vi "AM Init PS Scan.vi"(8 "error in (no error)":errorcluster, 10 "Message Data":variant, 11 "Hardware Resources in":T1 {"PS Measure Plan" items=["Pretreatment settings (PS)", "Linear Sweep Voltammetry (LSV)", "Differential Pulse Voltammetry (DPV)", "Cyclic Voltammetry (CV)", "Chronoamperometry (CA)", "Chronopotentiometry (CP)", "El Imp Spectroscopy (EIS)"]; "System Preset"."Test Configuration"."SP List" format="%#.1g"}) -> (0 "error out":errorcluster, 3 "Hardware Resources out":T1 {"PS Measure Plan" items=["Pretreatment settings (PS)", "Linear Sweep Voltammetry (LSV)", "Differential Pulse Voltammetry (DPV)", "Cyclic Voltammetry (CV)", "Chronoamperometry (CA)", "Chronopotentiometry (CP)", "El Imp Spectroscopy (EIS)"]; "System Preset"."Test Configuration"."SP List" format="%#.1g"})   [LabVIEW 2020, in "Test Driver.lvlib"]
doc: "Initialize the hardware references."
uses:
  Test Driver.lvlib
  Test Driver Configuration.ctl
  support/Message Queue/Message Cluster.ctl
  System Preset.ctl
  Test Type.ctl
  support/Message Queue/Message Queue.lvlib
panel:
  # "X"
  # "Y"
  # "Cycles"
  # "Point Delay"
  # "Up"
  # "Down"
  # "Z Axes"
  # "#C"
  # "In"
  # "Out"
  # "Cleaning [sec]"
  # "X"
  # "Y"
  # "Cycles"
  # "Point Delay"
  # "Up"
  # "Down"
  # "Z Axes"
  # "#C"
  # "In"
  # "Out"
  # "Cleaning [sec]"
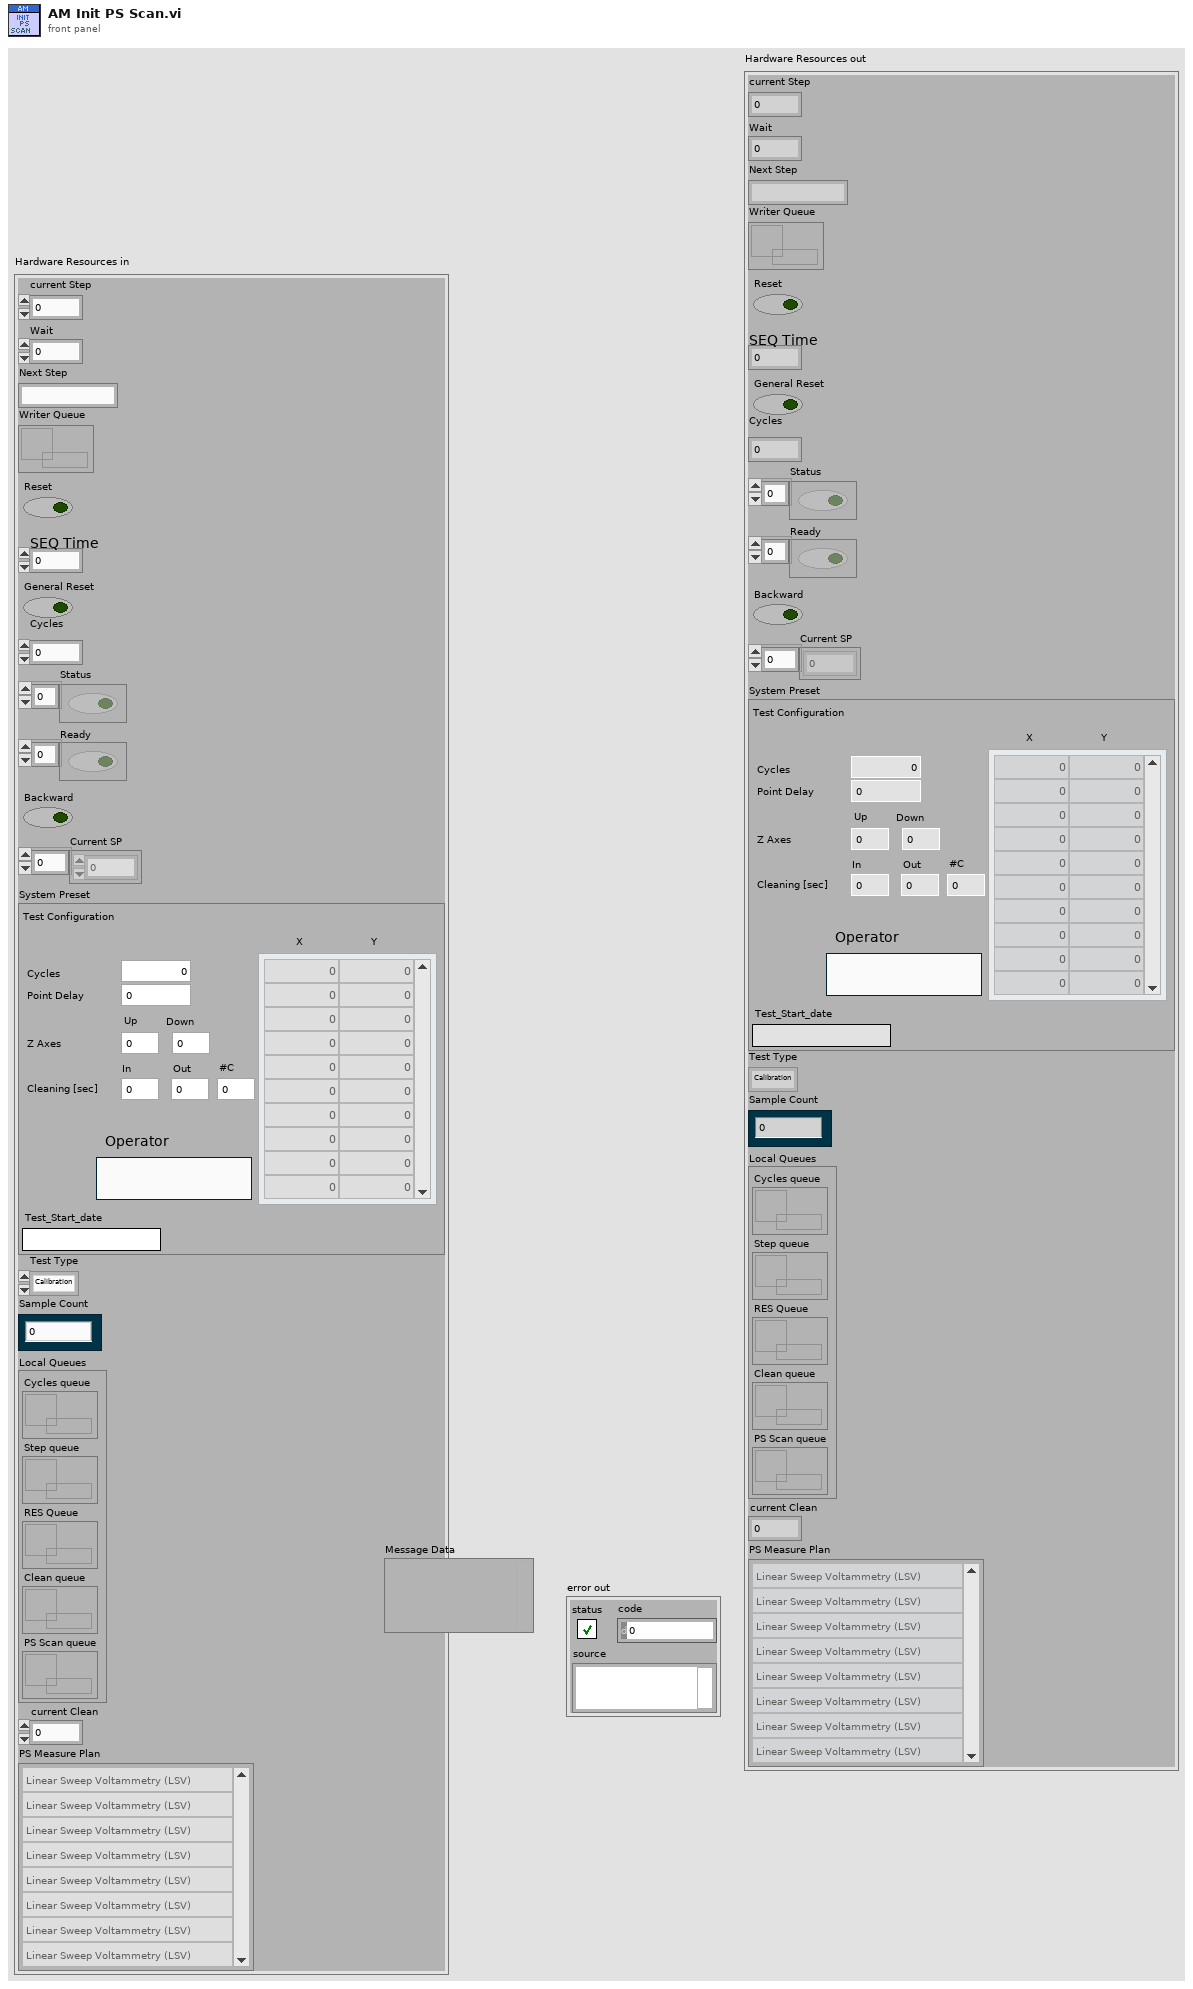
[diagram p1: front panel]
types:
  T1 = typedef "Test Driver.lvlib/Test Driver Configuration.ctl" = cluster{"current Step":i32, "Wait":dbl, "Next Step":string, "Writer Queue":refnum<queue>, "Reset":bool, "SEQ Time":i32, "General Reset":bool, "Cycles":i32, "Status":bool[], "Ready":bool[], "Backward":bool, "Current SP":dbl[], "System Preset":T2, "Test Type":T3, "Sample Count":i32, "Local Queues":cluster{"Cycles queue":refnum<queue>, "Step queue":refnum<queue>, "RES Queue":refnum<queue>, "Clean queue":refnum<queue>, "PS Scan queue":refnum<queue>}, "current Clean":i32, "PS Measure Plan":u16[]}
  T2 = typedef "System Preset.ctl" = cluster{"Test Configuration":cluster{"Cycles":i32, "Z Up":dbl, "SP List":dbl[][], "Operator":string, "Point Delay":i32, "Z Up 2":dbl, "Cleaning In":dbl, "Cleaning Out":dbl, "Cleaning Cycles":i32}, "Test_Start_date":string}
  T3 = typedef "Test Driver.lvlib/Test Type.ctl" = enum16{"Calibration", "Test"}
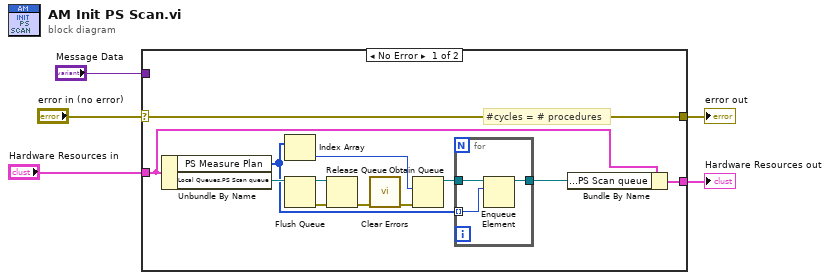
[diagram p0: block diagram]
diagram:
  n1 = case shown="No Error" "error in (no error)" {
    selector: "error in (no error)" -> [w15 w21]
    tunnel: [w15 w21] -> w4
    tunnel: "Hardware Resources in" -> [w16 w22]
    tunnel: [w17 w22] -> w1
    tunnel: "Message Data" -> [_ _]
    frame No Error {
      # "#cycles = # procedures"
      n2 = Unbundle By Name(w16) -> ("PS Measure Plan"=w6:u16[], "Local Queues.PS Scan queue"=w13:refnum<queue>)
      n3 = Index Array(array=w6) -> (element=w7:u16)  [unwired: 1 in]
      n4 = Flush Queue(queue=w13) -> (queue out=w10:refnum<queue>, error out=w11:errorcluster)  [unwired: 1 in, 1 out]
      n5 = Release Queue(queue=w10, error in (no error)=w11) -> (error out=w9:errorcluster)  [unwired: 1 in, 2 out]
      n6 = call <vilib>:"Clear Errors.vi"("error in (no error)"=w9) -> ("error out"=w14:errorcluster)  [unwired: 5 in, 1 out]
      n7 = Obtain Queue(element data type=w7, error in (no error)=w14) -> (queue out=w12:refnum<queue>)  [unwired: 3 in, 2 out]
      n8 = for {
        tunnel: w12 -> [w19]
        tunnel: [w20] -> w8
        tunnel: w6 -> [w18] mode=indexing
        n9 = Enqueue Element(queue=w19, element=w18) -> (queue out=w20:refnum<queue>)  [unwired: 2 in, 2 out]
      }
      n10 = Bundle By Name(cluster=w16, "Local Queues.PS Scan queue"=w8) -> (w17:T1)
    }
    frame Error {
    }
  }
  "Hardware Resources out" <- w1
  "error out" <- w4
